vi "SQL_test_template_data_deletebytempNo.vi"(11 "tempNo":string) -> (3 "error out":errorcluster)   [LabVIEW 2014]
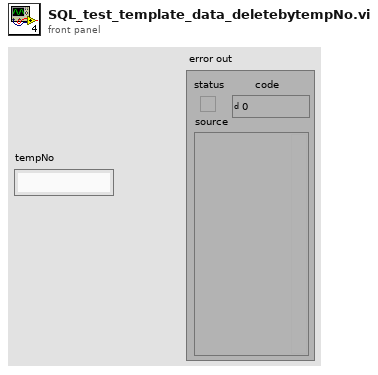
[diagram p1: front panel]
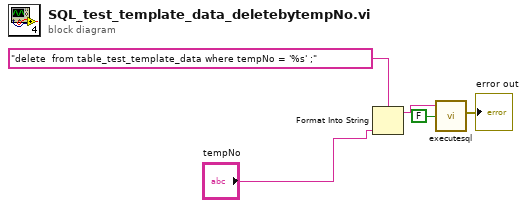
[diagram p0: block diagram]
diagram:
  n1 = Format Into String(format string="delete  from table_test_template_data where tempNo = '%s' ;" ("Command Text"), "tempNo") -> (resulting string=w3:string)  [unwired: 2 in, 1 out]
  n2 = call "executesql.vi"("Return Data (T)"=FALSE, "Command Text"=w3) -> ("error out"=→"error out":errorcluster)  [unwired: 5 in, 1 out]
